vi "New.vi"(6 "Node ID":u32, 8 "error in (no error)":errorcluster, 9 "Event Log Folder":path, 10 "Parent":refnum<class "Config Element.lvclass">, 11 "Name":string) -> (0 "error out":errorcluster, 3 "Node out":refnum<class "Node.lvclass">)   [LabVIEW 2020, in "VolatusConfig.lvlib" / "Node.lvclass"]
uses:
  Node.lvclass
  C:/dev/lv20CE/relink/lv-volatus/VolatusConfig/VolatusConfigElement/VolatusConfigElement.lvclass
  lv-cdm/CDM-Config/Config Element/Config Element.lvclass
  Meta Type.ctl
  lv-cdm/CDM-Config/Value Type.ctl
  Node.lvclass/Node.ctl
  lv-cdm/CDM-Config/CDM-Config.lvlib
  VolatusConfig.lvlib
  VolatusConfigElement/VolatusConfigElement.lvclass
  C:/dev/lv20CE/relink/lv-volatus/VolatusConfig/Node/Node.lvclass
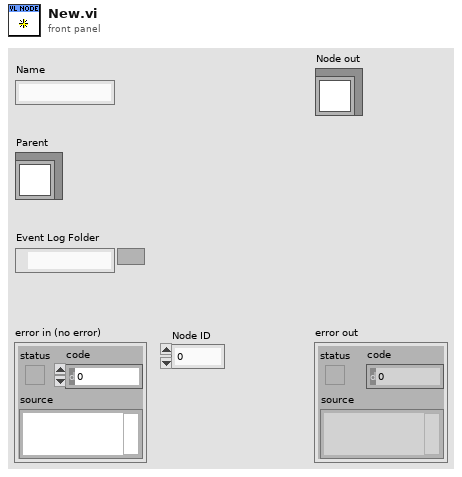
[diagram p1: front panel]
types:
  T1 = typedef "VolatusConfig.lvlib/Meta Type.ctl" = enum16{"UNKNOWN", "VL_System", "VL_Cluster", "VL_Node", "VL_Task", "VL_Group", "VL_Channel", "VL_Task_List", "VL_Scaling", "VL_Sensor", "VL_Sensor_List", "VL_Scale"}
  T2 = typedef "CDM-Config.lvlib/Value Type.ctl" = enum16{"String", "Number", "Bool", "Object", "Array"}
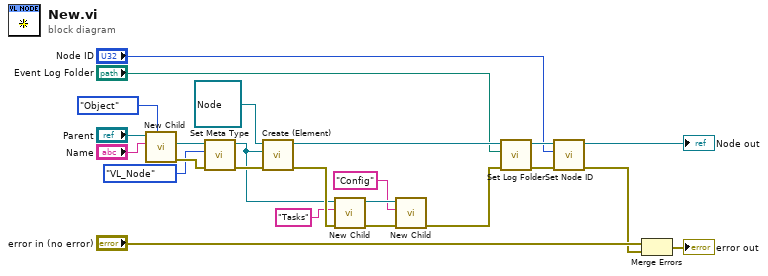
[diagram p0: block diagram]
diagram:
  n1 = call "New Child.vi"("Value Type (Object)"=Value_Type."Object" ("Value Type (String)"), "Child Name"="Name", "Config Element in"="Parent") -> ("error out"=w23:errorcluster, "New Child"=w18:refnum<class "Config Element.lvclass">)  [unwired: 6 in, 1 out]
  n2 = call "Set Meta Type.vi"("error in (no error)"=w23, "Meta Type"=Meta_Type."VL_Node", "Element In"=w18) -> ("error out"=w13:errorcluster, "Element"=w12:refnum<class "Config Element.lvclass">)  [unwired: 7 in]
  n3 = call "Create (Element).vi"("error in (no error)"=w13, "Element"=w12, "VolatusConfigElement in"=refnum<class "Node.lvclass"> refnum ("Node in")) -> ("error out"=w24:errorcluster, "VolatusConfigElement out"=w15:refnum<class "Node.lvclass">)  [unwired: 7 in]
  n4 = call "New Child.vi"("error in (no error)"=w24, "Child Name"="Tasks", "Config Element in"=w12) -> ("error out"=w3:errorcluster, "Config Element out"=w4:refnum<class "Config Element.lvclass">)  [unwired: 6 in, 1 out]
  n5 = call "New Child.vi"("error in (no error)"=w3, "Child Name"="Config", "Config Element in"=w4) -> ("error out"=w2:errorcluster)  [unwired: 6 in, 2 out]
  n6 = call "Set Log Folder.vi"("error in (no error)"=w2, "LogFolder"="Event Log Folder", "Node in"=w15) -> ("error out"=w9:errorcluster, "Node out"=w7:refnum<class "Node.lvclass">)  [unwired: 7 in]
  n7 = call "Set Node ID.vi"("error in (no error)"=w9, "Node ID"="Node ID", "Node in"=w7) -> ("error out"=w8:errorcluster, "Node out"=→"Node out":refnum<class "Node.lvclass">)  [unwired: 7 in]
  n8 = Merge Errors("error in (no error)", w8) -> (→"error out":errorcluster)
